vi "Init Tx - Data.vi"(7 "Data Access in":refnum<class "Data Access Engine.lvclass">, 8 "error in (no error)":errorcluster, 11 "Parameters":variant) -> (0 "error out":errorcluster, 3 "Tx Loop Data":T2, 5 "Data Access out":refnum<class "Data Access Engine.lvclass">)   [LabVIEW 2019, in "UDP-Custom-Device Engine.lvlib"]
uses:
  UDP-Custom-Device Engine.lvlib
  <vilib>/NI/NIVS Inline Async API/_Data Access Engine/Data Access Engine/Data Access Engine.lvclass
  Types/Engine - Tx Loop Data.ctl
  <vilib>/NI VeriStand/VeriStand Data/Byte Buffer/Byte Buffer.lvclass
  Types/Engine - General Resources.ctl
  <vilib>/NI VeriStand/VeriStand Data/Typedefs/Typedefs.Data Types.ctl
  Shared/Types/Shared - Duplex Settings.ctl
  Shared/Types/Shared - Header Details.ctl
  Types/Engine - Data Conversion Config.ctl
  <vilib>/NI VeriStand/VeriStand Data/Byte Buffer/Byte Buffer.Mapping.ctl
  Types/Engine - Tx Runtime Resources.ctl
  Shared/Types/Shared - Transmit Flag Options.ctl
  Types/Engine - Execution Config.ctl
  Shared/Types/Shared - Thread Management.ctl
  Types/Engine - Tx Echo Resources.ctl
  Shared/Types/Shared - Transmit Echo Options.ctl
  Types/Engine - Tx Channel Refs.ctl
  <vilib>/NI/NIVS Inline Async API/_Data Access Engine/Data Access Engine/Types/Read.DVR.ctl
  <vilib>/NI/NIVS Inline Async API/_Data Access Engine/Access Type Classes/Read/Read.lvclass
  <vilib>/NI/NIVS Inline Async API/_Data Access Engine/Data Access Engine/Types/Write.DVR.ctl
  <vilib>/NI/NIVS Inline Async API/_Data Access Engine/Access Type Classes/Write/Write.lvclass
  Types/Engine - Debug Resources.ctl
  Shared/Types/Shared - Channel Data Type.ctl
  Shared/Types/Shared - Tx.PacketInfo.ctl
  Shared/Types/Shared - Transmit Sim Options.ctl
  Shared/Types/Shared - Buffered.PacketInfo.ctl
  Shared/Types/Shared - Pointer Encoding.ctl
  Shared/Types/Shared - Receive Buffer Options.ctl
  Shared/Types/Shared - Transmit Buffer Options.ctl
  <vilib>/NI/NIVS Inline Async API/_Data Access Engine/Data Access Engine/Methods/Read.Lookup.vi
  <vilib>/NI/NIVS Inline Async API/_Data Access Engine/Data Access Engine/Methods/Write.Lookup.vi
  Shared/UDP-Custom-Device Shared.lvlib
  <vilib>/NI VeriStand/VeriStand Data/VeriStand Data.lvlib
panel:
  out "Channel Data Types":T1[](array[typedef])
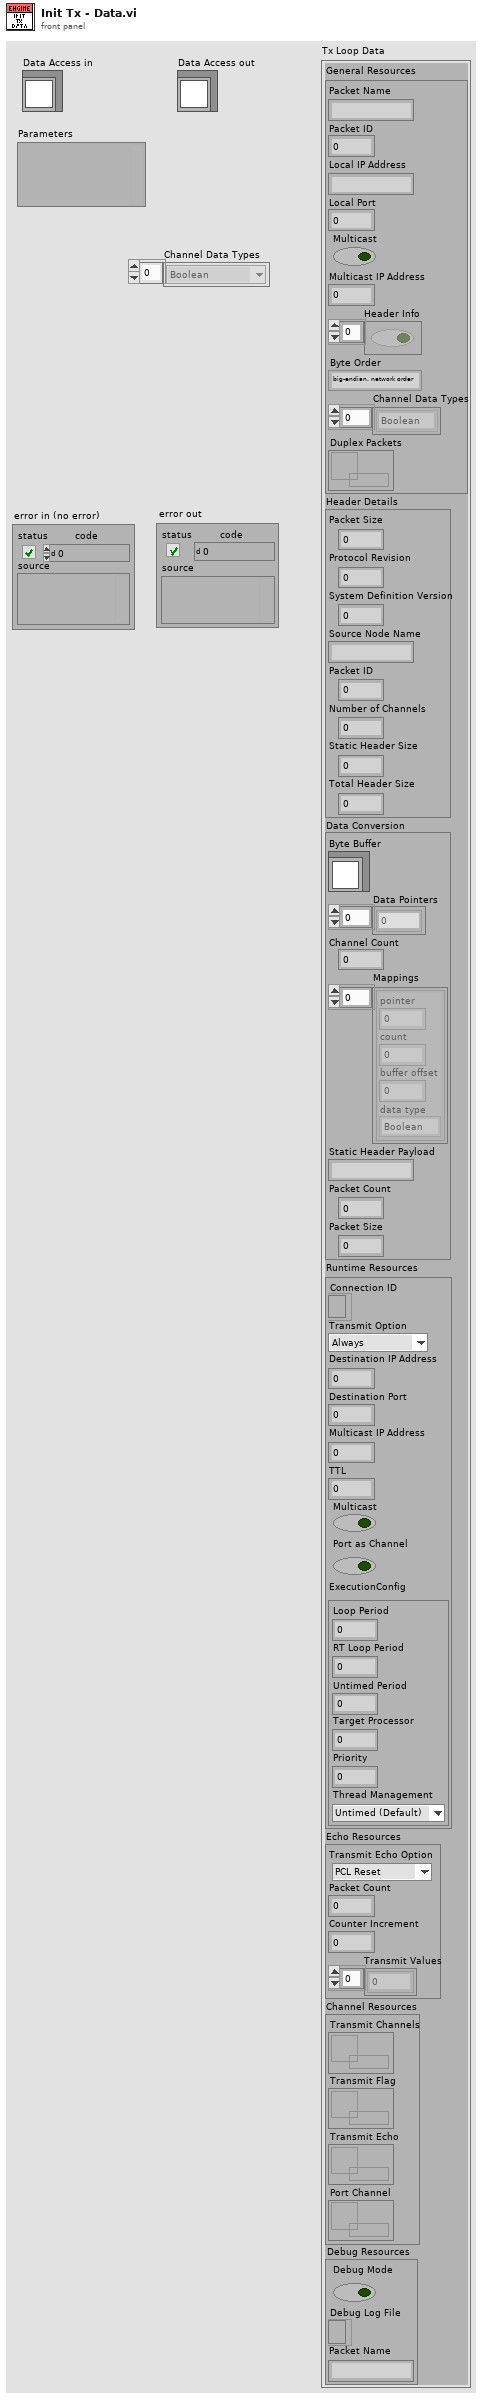
[diagram p1: front panel]
types:
  T1 = typedef "UDP-Custom-Device Shared.lvlib/Shared - Channel Data Type.ctl" = enum16{"Boolean", "Single", "Double", "I8", "I16", "I32", "I64", "U8", "U16", "U32", "U64"}
  T2 = typedef "UDP-Custom-Device Engine.lvlib/Engine - Tx Loop Data.ctl" = cluster{"General Resources":T3, "Header Details":T5, "Data Conversion":T6, "Runtime Resources":T8, "Echo Resources":T12, "Channel Resources":T14, "Debug Resources":T17}
  T3 = typedef "UDP-Custom-Device Engine.lvlib/Engine - General Resources.ctl" = cluster{"Packet Name":string, "Packet ID":i32, "Local IP Address":string, "Local Port":i32, "Multicast":bool, "Multicast IP Address":u32, "Header Info":bool[], "Byte Order":enum16{"big-endian, network order", "native, host order", "little-endian"}, "Channel Data Types":T4[], "Duplex Packets":refnum<data-value>}
  T4 = typedef "VeriStand Data.lvlib/Typedefs.Data Types.ctl" = enum16{"Boolean", "Single", "Double", "I8", "I16", "I32", "I64", "U8", "U16", "U32", "U64"}
  T5 = typedef "UDP-Custom-Device Shared.lvlib/Shared - Header Details.ctl" = cluster{"Packet Size":u16, "Protocol Revision":u8, "System Definition Version":u64, "Source Node Name":string, "Packet ID":u32, "Number of Channels":u32, "Static Header Size":u16, "Total Header Size":u16}
  T6 = typedef "UDP-Custom-Device Engine.lvlib/Engine - Data Conversion Config.ctl" = cluster{"Byte Buffer":refnum<class "Byte Buffer.lvclass">, "Data Pointers":u64[], "Channel Count":i32, "Mappings":T7[], "Static Header Payload":string, "Packet Count":dbl, "Packet Size":i32}
  T7 = typedef "VeriStand Data.lvlib/Byte Buffer.lvclass/Byte Buffer.Mapping.ctl" = cluster{"pointer":u64, "count":i64, "buffer offset":u64, "data type":T4}
  T8 = typedef "UDP-Custom-Device Engine.lvlib/Engine - Tx Runtime Resources.ctl" = cluster{"Connection ID":refnum<k16>, "Transmit Option":T9, "Destination IP Address":u32, "Destination Port":u16, "Multicast IP Address":u32, "TTL":u16, "Multicast":bool, "Port as Channel":bool, "ExecutionConfig":T10}
  T9 = typedef "UDP-Custom-Device Shared.lvlib/Shared - Transmit Flag Options.ctl" = enum16{"Always", "One-Shot", "Toggle"}
  T10 = typedef "UDP-Custom-Device Engine.lvlib/Engine - Execution Config.ctl" = cluster{"Loop Period":i64, "RT Loop Period":i64, "Untimed Period":u32, "Target Processor":i32, "Priority":i32, "Thread Management":T11}
  T11 = typedef "UDP-Custom-Device Shared.lvlib/Shared - Thread Management.ctl" = enum16{"Untimed (Default)", "Timed (High Priority)"}
  T12 = typedef "UDP-Custom-Device Engine.lvlib/Engine - Tx Echo Resources.ctl" = cluster{"Transmit Echo Option":T13, "Packet Count":dbl, "Counter Increment":dbl, "Transmit Values":dbl[]}
  T13 = typedef "UDP-Custom-Device Shared.lvlib/Shared - Transmit Echo Options.ctl" = enum16{"PCL Reset", "Counter", "Mirror"}
  T14 = typedef "UDP-Custom-Device Engine.lvlib/Engine - Tx Channel Refs.ctl" = cluster{"Transmit Channels":T15, "Transmit Flag":T15, "Transmit Echo":T16, "Port Channel":T15}
  T15 = typedef "Data Access Engine.lvlib/Data Access Engine.lvclass/Read.DVR.ctl" = refnum<data-value>
  T16 = typedef "Data Access Engine.lvlib/Data Access Engine.lvclass/Write.DVR.ctl" = refnum<data-value>
  T17 = typedef "UDP-Custom-Device Engine.lvlib/Engine - Debug Resources.ctl" = cluster{"Debug Mode":bool, "Debug Log File":refnum<file>, "Packet Name":string}
  T18 = typedef "UDP-Custom-Device Shared.lvlib/Shared - Tx.PacketInfo.ctl" = cluster{"Packet Name":string, "Packet ID":i32, "Decimation":u16, "Destination IP Address":string, "Destination Port":u16, "Local IP Address":string, "Local Port":u16, "Endianness":u16, "TTL":u16, "Multicast":bool, "Multicast IP Address":string, "Transmit Option":T9, "Transmit Echo Option":T13, "Transmit Sim Option":T19, "Port as Channel":bool, "Debug Mode":bool, "Header Info":bool[], "Loop Period":u32, "Channel Data Types":T1[], "Header Details":T5, "Buffered Packet Info":T20, "Duplex Packets":refnum<data-value>, "targetProcessor":i8, "targetPriority":i16, "Thread Management":T11}
  T19 = typedef "UDP-Custom-Device Shared.lvlib/Shared - Transmit Sim Options.ctl" = enum16{"No Simulation", "Counter", "Full Buffer", "FIFO Test", "FIFO + Port Test"}
  T20 = typedef "UDP-Custom-Device Shared.lvlib/Shared - Buffered.PacketInfo.ctl" = cluster{"Buffer Size":i32, "External Buffer":bool, "Prepend Header":bool, "Is Buffered":bool, "Pointer Encoding":T21, "Rx Buffer Option":T22, "Tx Buffer Option":T23}
  T21 = typedef "UDP-Custom-Device Shared.lvlib/Shared - Pointer Encoding.ctl" = enum16{"Direct Encoding", "Conversion Encoding"}
  T22 = typedef "UDP-Custom-Device Shared.lvlib/Shared - Receive Buffer Options.ctl" = enum16{"Static Buffer", "Circular Buffer", "Circular Buffer + Size", "Internal Cache", "Internal Cache + Size", "Ping Pong", "Ping Pong + Size"}
  T23 = typedef "UDP-Custom-Device Shared.lvlib/Shared - Transmit Buffer Options.ctl" = enum16{"Static Buffer", "FIFO Buffer", "FIFO Buffer + Port"}
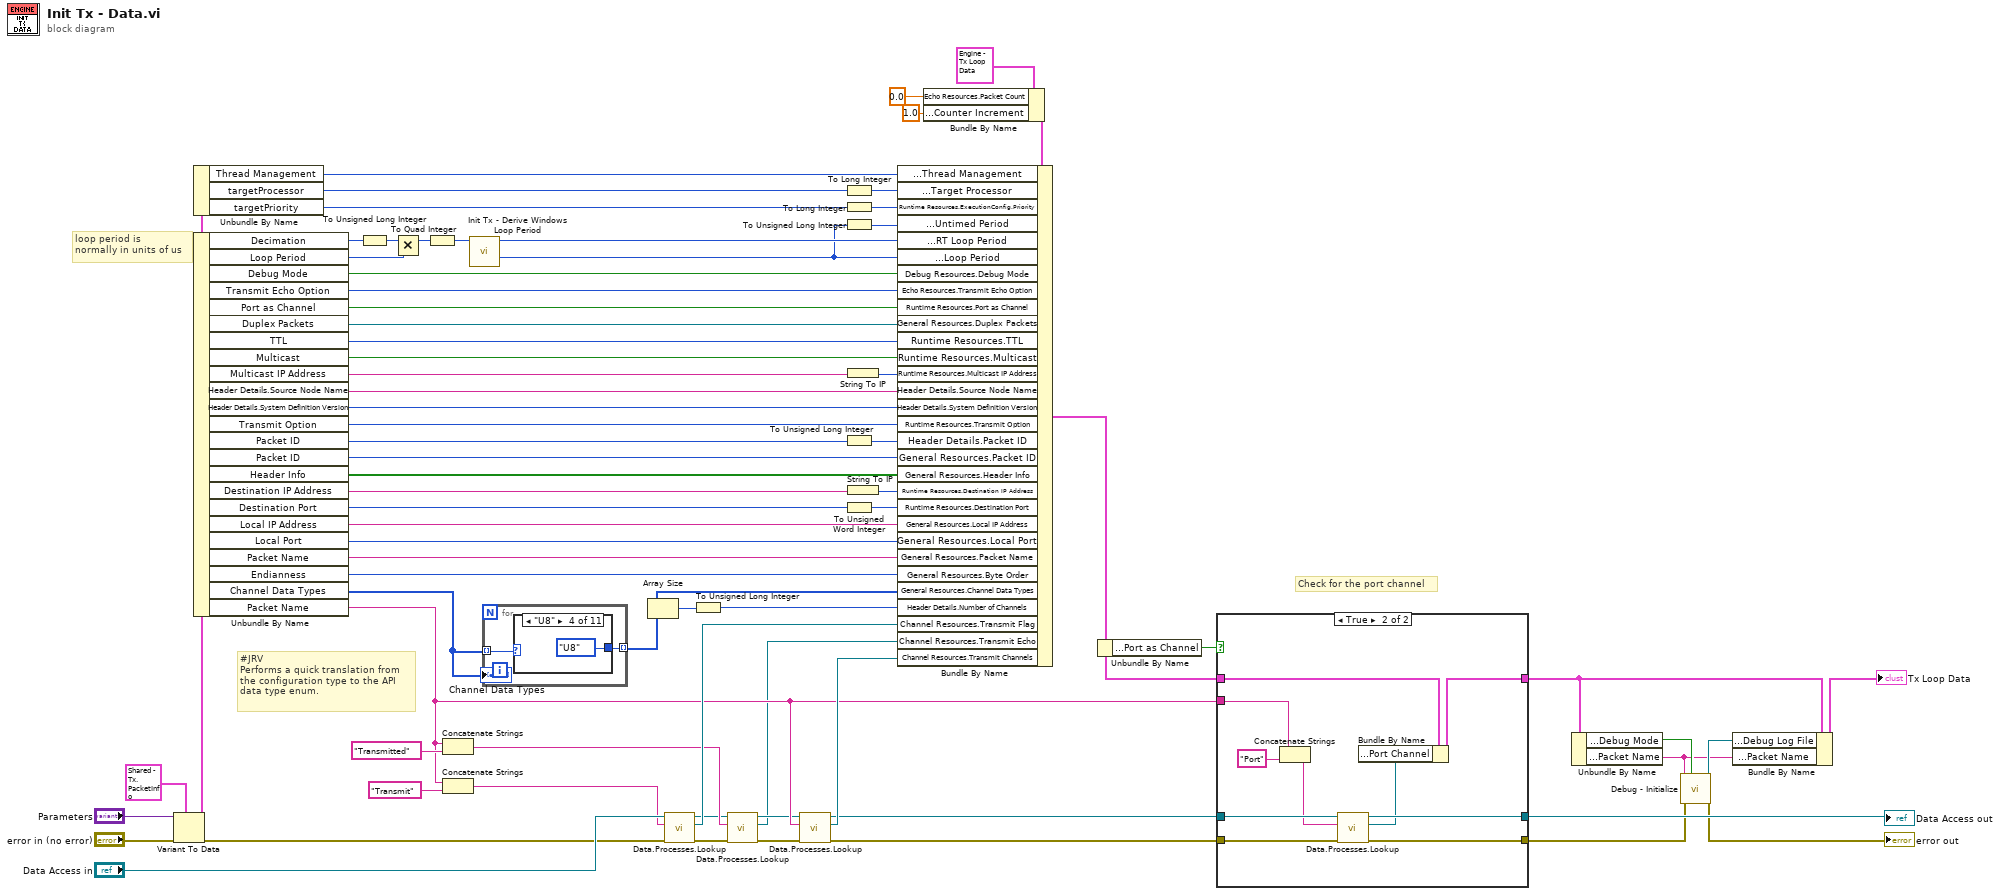
[diagram p0: block diagram]
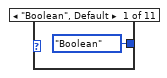
[diagram p2: hidden frame]
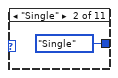
[diagram p3: hidden frame]
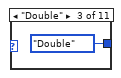
[diagram p4: hidden frame]
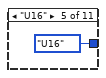
[diagram p5: hidden frame]
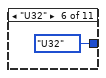
[diagram p6: hidden frame]
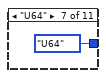
[diagram p7: hidden frame]
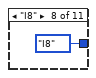
[diagram p8: hidden frame]
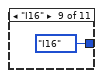
[diagram p9: hidden frame]
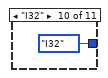
[diagram p10: hidden frame]
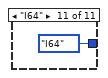
[diagram p11: hidden frame]
diagram:
  # "loop period is\nnormally in units of us"
  # "Check for the port channel"
  # "#JRV\nPerforms a quick translation from\nthe configuration type to the API\ndata type enum."
  n1 = Variant To Data(error in="error in (no error)", type=T18 {"Packet Name"="", "Packet ID"=0, "Decimation"=0, "Destination IP Address"="", "Destination Port"=0, "Local IP Address"="", "Local Port"=0, "Endianness"=0, "TTL"=0, "Multicast"=FALSE, "Multicast IP Address"="", "Transmit Option"=enum."Always", "Transmit Echo Option"=enum."PCL Reset", "Transmit Sim Option"=enum."No Simulation", "Port as Channel"=FALSE, "Debug Mode"=FALSE, "Header Info"=[], "Loop Period"=0, "Channel Data Types"=[], "Header Details"={"Packet Size"=0, "Protocol Revision"=0, "System Definition Version"=0, "Source Node Name"="", "Packet ID"=0, "Number of Channels"=0, "Static Header Size"=0, "Total Header Size"=0}, "Buffered Packet Info"={"Buffer Size"=0, "External Buffer"=FALSE, "Prepend Header"=FALSE, "Is Buffered"=FALSE, "Pointer Encoding"=enum."Direct Encoding", "Rx Buffer Option"=enum."Static Buffer", "Tx Buffer Option"=enum."Static Buffer"}, "Duplex Packets"=refnum, "targetProcessor"=0, "targetPriority"=1, "Thread Management"=enum."Untimed (Default)"} ("Packet Info"), Variant="Parameters") -> (data=w4:T18, error out=w51:errorcluster)
  n2 = Unbundle By Name(w4) -> ("Thread Management"=w3:T11, "targetProcessor"=w2:i8, "targetPriority"=w1:i16)
  n3 = Unbundle By Name(w4) -> ("Decimation"=w14:u16, "Loop Period"=w13:u32, "Debug Mode"=w27:bool, "Transmit Echo Option"=w28:T13, "Port as Channel"=w42:bool, "Duplex Packets"=w43:refnum<data-value>, "TTL"=w47:u16, "Multicast"=w46:bool, "Multicast IP Address"=w45:string, "Header Details.Source Node Name"=w54:string, "Header Details.System Definition Version"=w53:u64, "Transmit Option"=w66:T9, "Packet ID"=w59:i32, "Packet ID"=w12:i32, "Header Info"=w65:bool[], "Destination IP Address"=w61:string, "Destination Port"=w63:u16, "Local IP Address"=w70:string, "Local Port"=w69:u16, "Packet Name"=w71:string, "Endianness"=w67:u16, "Channel Data Types"=w64:T1[], "Packet Name"=w35:string)
  "Channel Data Types" <- w64
  n4 = To Unsigned Long Integer(number=w14) -> (unsigned 32bit integer=w15:u32)
  n5 = Multiply(x=w15, y=w13) -> (x*y=w11:u32)
  n6 = To Quad Integer(1:w11) -> (0:w10:i64)
  n7 = Concatenate Strings(w35, "Transmitted" ("Item GUID")) -> (w34:string)
  n8 = Concatenate Strings(w35, "Transmit" ("Item GUID")) -> (w49:string)
  n9 = call "Init Tx - Derive Windows Loop Period.vi"("RT Loop Period in"=w10) -> ("Win Loop Period out"=w5:i64, "RT Loop Period out"=w9:i64)  [unwired: 9 in]
  n10 = for {
    tunnel: w64 -> [w76] mode=indexing
    tunnel: [w75] -> w57 mode=indexing
    n11 = case shown="\"U8\"" w76 {
      tunnel: [Typedefs.Data_Types."Boolean" ("data type") Typedefs.Data_Types."Single" ("data type") Typedefs.Data_Types."Double" ("data type") Typedefs.Data_Types."U8" ("data type") Typedefs.Data_Types."U16" ("data type") Typedefs.Data_Types."U32" ("data type") Typedefs.Data_Types."U64" ("data type") Typedefs.Data_Types."I8" ("data type") Typedefs.Data_Types."I16" ("data type") Typedefs.Data_Types."I32" ("data type") Typedefs.Data_Types."I64" ("data type")] -> w75
      frame "Boolean", Default {
      }
      frame "Single" {
      }
      frame "Double" {
      }
      frame "U8" {
      }
      frame "U16" {
      }
      frame "U32" {
      }
      frame "U64" {
      }
      frame "I8" {
      }
      frame "I16" {
      }
      frame "I32" {
      }
      frame "I64" {
      }
    }
  }
  n12 = Array Size(array=w57) -> (size(s)=w56:i32)
  n13 = call-poly <vilib>:"Data.Processes.Lookup.vi"("error in (no error)"=w51, "Name"=w49, "Data Access API in"="Data Access in") -> ("error out"=w31:errorcluster, "Ref"=w48:T15, "Data Access API out"=w33:refnum<class "Data Access Engine.lvclass">)  [unwired: 5 in, 1 out]
  n14 = To Unsigned Long Integer(number=w56) -> (unsigned 32bit integer=w55:u32)
  n15 = call-poly <vilib>:"Data.Processes.Lookup.vi"("error in (no error)"=w31, "Name"=w34, "Data Access API in"=w33) -> ("error out"=w30:errorcluster, "Ref"=w29:T16, "Data Access API out"=w32:refnum<class "Data Access Engine.lvclass">)  [unwired: 5 in, 1 out]
  n16 = call-poly <vilib>:"Data.Processes.Lookup.vi"("error in (no error)"=w30, "Name"=w35, "Data Access API in"=w32) -> ("error out"=w39:errorcluster, "Ref"=w68:T15, "Data Access API out"=w41:refnum<class "Data Access Engine.lvclass">)  [unwired: 5 in, 1 out]
  n17 = To Long Integer(number=w2) -> (32bit integer=w8:i32)
  n18 = To Long Integer(number=w1) -> (32bit integer=w7:i32)
  n19 = To Unsigned Long Integer(number=w5) -> (unsigned 32bit integer=w6:u32)
  n20 = To Unsigned Long Integer(number=w59) -> (unsigned 32bit integer=w58:u32)
  n21 = To Unsigned Word Integer(number=w63) -> (unsigned 16bit integer=w62:u16)
  n22 = String To IP(1:w45) -> (0:w44:u32)
  n23 = String To IP(1:w61) -> (0:w60:u32)
  n24 = Bundle By Name(cluster=T2 {"General Resources"={"Packet Name"="", "Packet ID"=0, "Local IP Address"="", "Local Port"=0, "Multicast"=FALSE, "Multicast IP Address"=0, "Header Info"=[], "Byte Order"=enum."big-endian, network order", "Channel Data Types"=[], "Duplex Packets"=refnum}, "Header Details"={"Packet Size"=0, "Protocol Revision"=0, "System Definition Version"=0, "Source Node Name"="", "Packet ID"=0, "Number of Channels"=0, "Static Header Size"=0, "Total Header Size"=0}, "Data Conversion"={"Byte Buffer"=refnum, "Data Pointers"=[], "Channel Count"=0, "Mappings"=[], "Static Header Payload"="", "Packet Count"=0.0, "Packet Size"=0}, "Runtime Resources"={"Connection ID"=refnum, "Transmit Option"=enum."Always", "Destination IP Address"=0, "Destination Port"=0, "Multicast IP Address"=0, "TTL"=0, "Multicast"=FALSE, "Port as Channel"=FALSE, "ExecutionConfig"={"Loop Period"=0, "RT Loop Period"=0, "Untimed Period"=0, "Target Processor"=0, "Priority"=0, "Thread Management"=enum."Untimed (Default)"}}, "Echo Resources"={"Transmit Echo Option"=enum."PCL Reset", "Packet Count"=0.0, "Counter Increment"=0.0, "Transmit Values"=[]}, "Channel Resources"={"Transmit Channels"=refnum, "Transmit Flag"=refnum, "Transmit Echo"=refnum, "Port Channel"=refnum}, "Debug Resources"={"Debug Mode"=FALSE, "Debug Log File"=refnum, "Packet Name"=""}} ("Tx Loop Data"), "Echo Resources.Packet Count"=0.0, "Echo Resources.Counter Increment"=1.0) -> (w17:T2)
  n25 = Bundle By Name(cluster=w17, "Runtime Resources.ExecutionConfig.Thread Management"=w3, "Runtime Resources.ExecutionConfig.Target Processor"=w8, "Runtime Resources.ExecutionConfig.Priority"=w7, "Runtime Resources.ExecutionConfig.Untimed Period"=w6, "Runtime Resources.ExecutionConfig.RT Loop Period"=w9, "Runtime Resources.ExecutionConfig.Loop Period"=w5, "Debug Resources.Debug Mode"=w27, "Echo Resources.Transmit Echo Option"=w28, "Runtime Resources.Port as Channel"=w42, "General Resources.Duplex Packets"=w43, "Runtime Resources.TTL"=w47, "Runtime Resources.Multicast"=w46, "Runtime Resources.Multicast IP Address"=w44, "Header Details.Source Node Name"=w54, "Header Details.System Definition Version"=w53, "Runtime Resources.Transmit Option"=w66, "Header Details.Packet ID"=w58, "General Resources.Packet ID"=w12, "General Resources.Header Info"=w65, "Runtime Resources.Destination IP Address"=w60, "Runtime Resources.Destination Port"=w62, "General Resources.Local IP Address"=w70, "General Resources.Local Port"=w69, "General Resources.Packet Name"=w71, "General Resources.Byte Order"=w67, "General Resources.Channel Data Types"=w57, "Header Details.Number of Channels"=w55, "Channel Resources.Transmit Flag"=w48, "Channel Resources.Transmit Echo"=w29, "Channel Resources.Transmit Channels"=w68) -> (w37:T2)
  n26 = Unbundle By Name(w37) -> ("Runtime Resources.Port as Channel"=w38:bool)
  n27 = case shown="True" w38 {
    tunnel: w35 -> [_ w99]
    tunnel: w41 -> [w89 w98]
    tunnel: [w89 w97] -> w40
    tunnel: w39 -> [w88 w96]
    tunnel: [w88 w95] -> w21
    tunnel: w37 -> [w90 w94]
    tunnel: [w90 w91] -> w23
    frame False {
    }
    frame True {
      n28 = Concatenate Strings(w99, "Port" ("Item GUID")) -> (w92:string)
      n29 = call-poly <vilib>:"Data.Processes.Lookup.vi"("error in (no error)"=w96, "Name"=w92, "Data Access API in"=w98) -> ("error out"=w95:errorcluster, "Ref"=w93:T15, "Data Access API out"=w97:refnum<class "Data Access Engine.lvclass">)  [unwired: 5 in, 1 out]
      n30 = Bundle By Name(cluster=w94, "Channel Resources.Port Channel"=w93) -> (w91:T2)
    }
  }
  "Data Access out" <- w40
  n31 = Unbundle By Name(w23) -> ("Debug Resources.Debug Mode"=w26:bool, "General Resources.Packet Name"=w20:string)
  n32 = call "Debug - Initialize.vi"("Debug Mode"=w26, "error in (no error)"=w21, "Packet Name"=w20) -> ("error out"=→"error out":errorcluster, "Debug Log File"=w25:refnum<file>)  [unwired: 7 in]
  n33 = Bundle By Name(cluster=w23, "Debug Resources.Debug Log File"=w25, "Debug Resources.Packet Name"=w20) -> (→"Tx Loop Data":T2)
